vi "trigger_front_pannel.vi"(6 "force close (F)":bool, 9 "error in (no error)":errorcluster, 10 "vi reference":refnum<vi>) -> (1 "error out":errorcluster, 2 "vi reference out":refnum<vi>, 4 "opened?":bool)   [LabVIEW 2015]
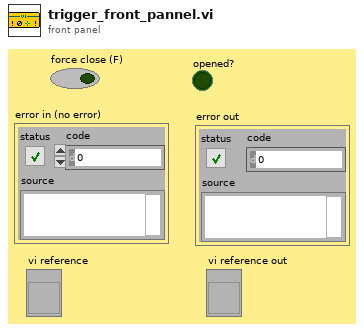
[diagram p1: front panel]
types:
  T1 = enum32{"Invalid", "Standard", "Closed", "Hidden", "Minimized", "Maximized"}
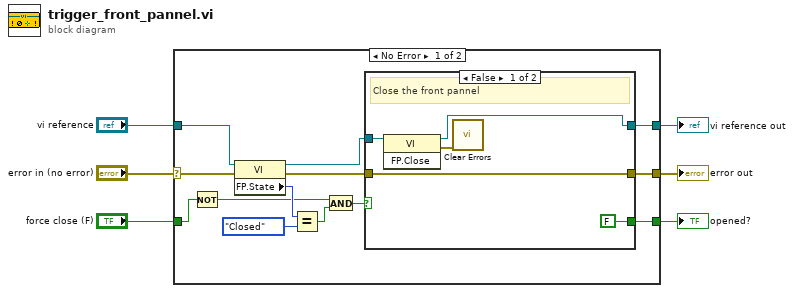
[diagram p0: block diagram]
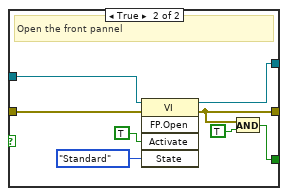
[diagram p2: hidden frame]
diagram:
  n1 = case shown="No Error" "error in (no error)" {
    selector: "error in (no error)" -> [w16 w34]
    tunnel: [w19 w34] -> w6
    tunnel: "force close (F)" -> [w18 _]
    tunnel: [w17 _] -> w4
    tunnel: "vi reference" -> [w8 w33]
    tunnel: [w7 w33] -> w1
    frame No Error {
      n2 = Not(x=w18) -> (.not. x?=w11:bool)
      n3 = property class="VI"(reference=w8, error in=w16) -> (reference out=w15:refnum<vi>, error out=w12:errorcluster, "FP.State"=w14:T1)
      n4 = Equal?(x=w14, y=T1."Closed") -> (x = y?=w10:bool)
      n5 = And(x=w11, y=w10) -> (x .and. y?=w9:bool)
      n6 = case shown="False" w9 {
        tunnel: w15 -> [w24 w30]
        tunnel: [w22 w29] -> w7
        tunnel: w12 -> [w21 w28]
        tunnel: [w21 w26] -> w19
        tunnel: [FALSE w25] -> w17
        frame False {
          # "Close the front pannel"
          n7 = invoke class="VI" method="FP.Close"(reference=w24) -> (reference out=w22:refnum<vi>, error out=w23:errorcluster)  [unwired: 2 in, 1 out]
          n8 = call <vilib>:"Clear Errors.vi"("error in (no error)"=w23) -> ()  [unwired: 5 in, 2 out]
        }
        frame True {
          # "Open the front pannel"
          n9 = invoke class="VI" method="FP.Open"(reference=w30, error in=w28, "Activate"=TRUE ("Activate?"), "State"=T1."Standard") -> (reference out=w29:refnum<vi>, error out=w26:errorcluster)  [unwired: 1 in, 3 out]
          n10 = And(x=w26, y=TRUE) -> (x .and. y?=w25:bool)
        }
      }
    }
    frame Error {
    }
  }
  "opened?" <- w4
  "error out" <- w6
  "vi reference out" <- w1
